vi "D_Datagrid example.vi"(10 "Remote stop event":refnum<user-event>, 11 "Owning VI":refnum<vi>) -> ()   [LabVIEW 2023, in "D Datagrid Library.lvlib"]
uses:
  D Datagrid Library.lvlib
  Scrolling behavior.ctl
  U32 D Element/U32 D Element.lvclass
  U8 D Element/U8 D Element.lvclass
  Bool D Element/Bool D Element.lvclass
  U32 D Element/Display mode.ctl
  String Dropdown D Element/String dropdown D Element.lvclass
  COM port D Element/COM Port D Element.lvclass
  D_Datagrid.lvclass
  String D Element/String D Element.lvclass
  String Dropdown D Element/String dropdown D Element.lvclass/String dropdown D Element.ctl
  U8 D Element/U8 D Element.lvclass/U8 D Element.ctl
  String D Element/String D Element.lvclass/String D Element.ctl
  DatagridElement/DatagridElement.lvclass/DatagridElement.ctl
  Bool D Element/Bool D Element.lvclass/Bool D Element.ctl
  D_Datagrid.lvclass/D_Datagrid.ctl
  Write Auto update indicator.vi
  Bool D Element/Write F string.vi
  Bool D Element/Write T string.vi
  String Dropdown D Element/Write value.vi
  String Dropdown D Element/Write Strings.vi
  U8 D Element/Write Display mode.vi
  String D Element/Write Value.vi
  DatagridElement/Write Enabled state.vi
  Read Auto update indicator.vi
  DatagridElement/DatagridElement.lvclass
  C:/dev/D Datagrid/DatagridElement/DatagridElement.lvclass
  C:/dev/D Datagrid/String D Element/String D Element.lvclass
  C:/dev/D Datagrid/Bool D Element/Bool D Element.lvclass
  C:/dev/D Datagrid/U32 D Element/U32 D Element.lvclass
  C:/dev/D Datagrid/U8 D Element/U8 D Element.lvclass
  C:/dev/D Datagrid/String Dropdown D Element/String dropdown D Element.lvclass
  C:/dev/D Datagrid/COM port D Element/COM Port D Element.lvclass
panel:
  in  "Scrolling mode":T1
  in  "Update now":bool
  in  "Auto-update?":bool=TRUE
  out "New?":bool
  out "Data as string":string
  out "Column":i32
  out "Row":i32
  in  "Datagrid table":string[][](table)
  # "This is an optional input\nused if this VI is to be\ncalled from within a\nsubpanel."
  # "This event stops\nthe VI (if used\nin subpanel)"
  # "Element touched"
  # "Instructions:\n1- Run the VI.\n2- Click each cell. Disabled string and Grayed string\n     cannot be edited, but the rest can.\n3. Observe the Element Touched event information."
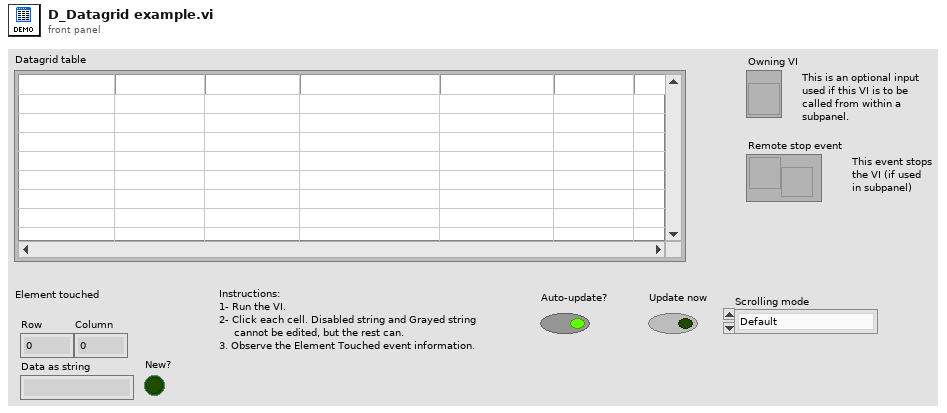
[diagram p1: front panel]
types:
  T1 = typedef "D Datagrid Library.lvlib/D_Datagrid.lvclass/Scrolling behavior.ctl" = enum16{"Default", "Locked", "Displayed items only"}
  T2 = enum8{"Enabled", "Disabled", "Disabled and Grayed Out"}
  T3 = typedef "D Datagrid Library.lvlib/U32 D Element.lvclass/Display mode.ctl" = enum16{"Standard", "Hex"}
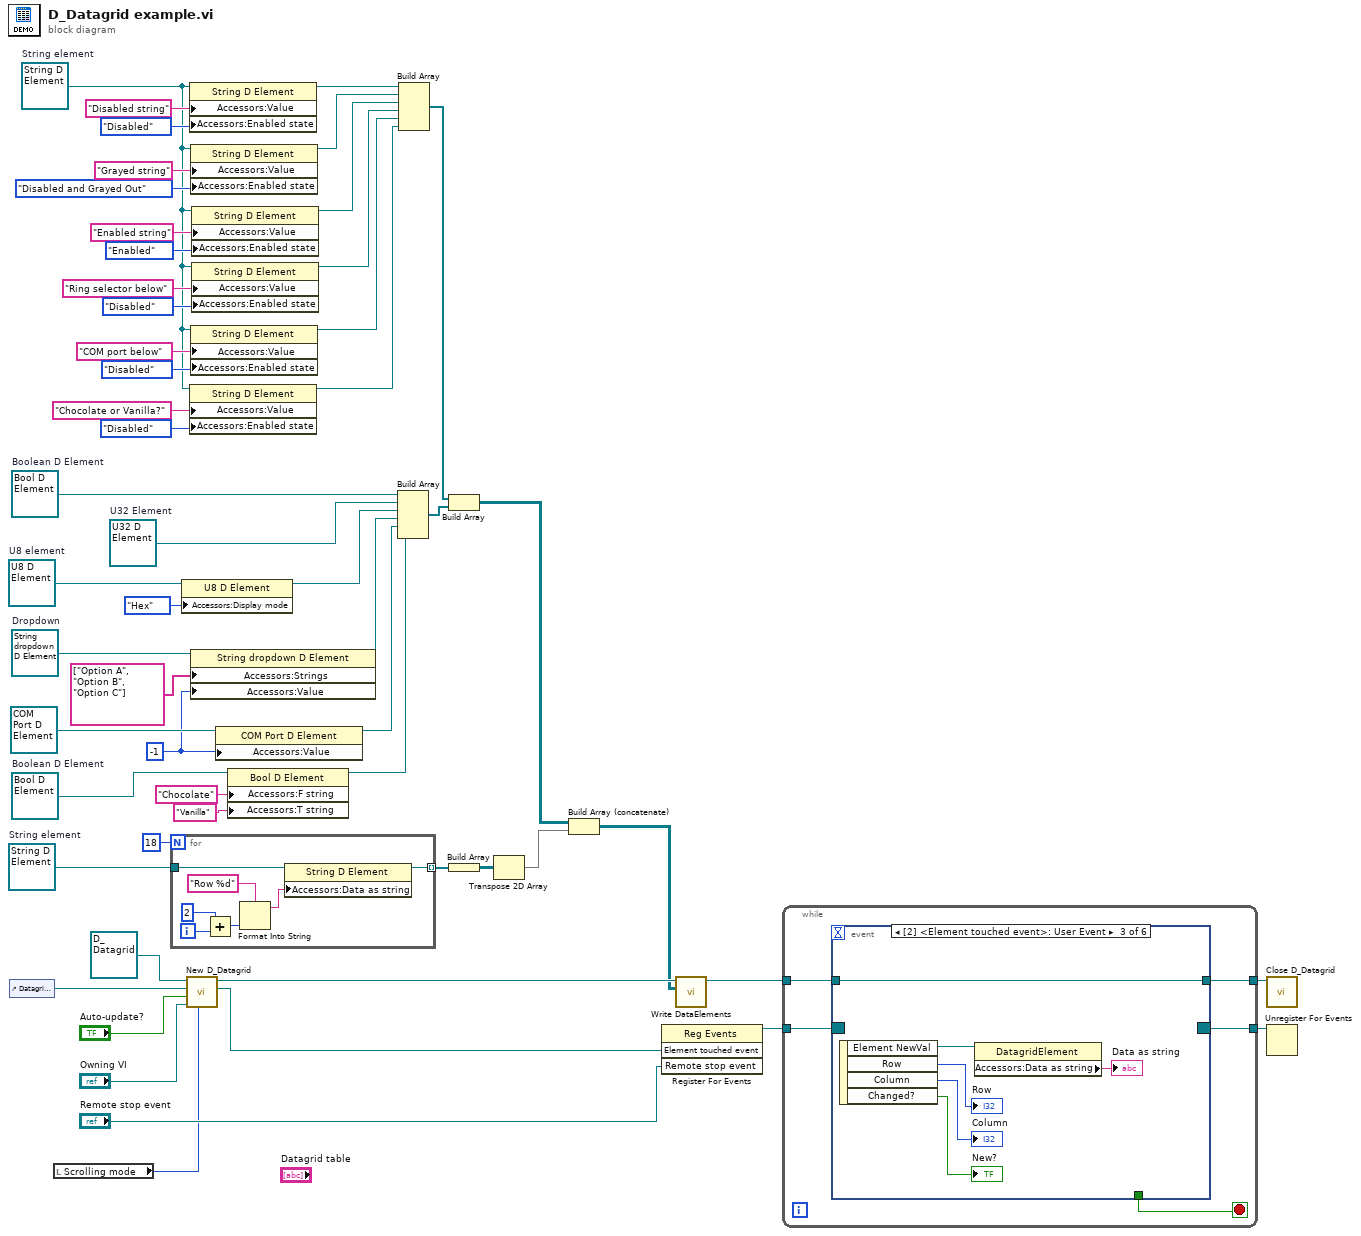
[diagram p0: block diagram]
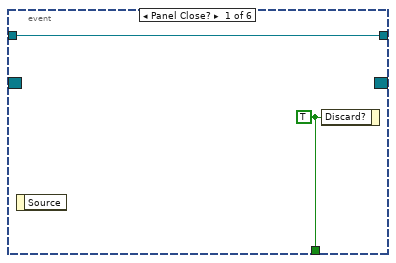
[diagram p2: hidden frame]
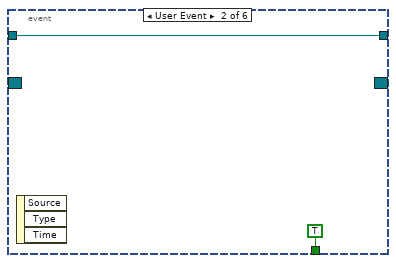
[diagram p3: hidden frame]
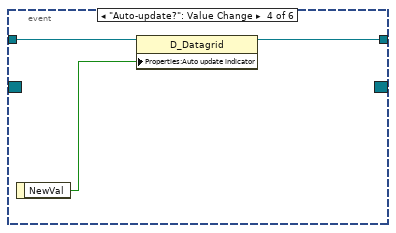
[diagram p4: hidden frame]
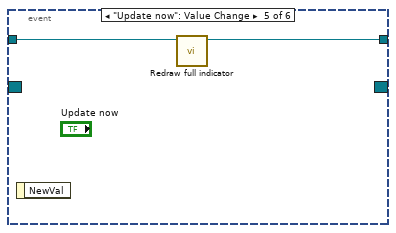
[diagram p5: hidden frame]
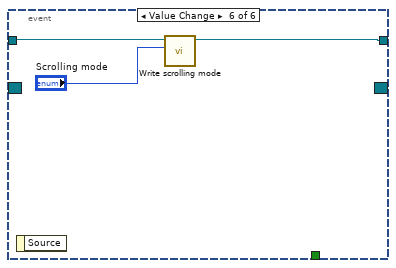
[diagram p6: hidden frame]
diagram:
  w8 = refnum<class "String D Element.lvclass"> refnum  # String element
  w14 = refnum<class "Bool D Element.lvclass"> refnum  # Boolean D Element
  w21 = -1 ("Value")
  w29 = refnum<class "String dropdown D Element.lvclass"> refnum  # Dropdown
  w38 = refnum<class "Bool D Element.lvclass"> refnum  # Boolean D Element
  w40 = refnum<class "U8 D Element.lvclass"> refnum  # U8 element
  w37 = refnum<class "U32 D Element.lvclass"> refnum  # U32 Element
  w9 = refnum<class "String D Element.lvclass"> refnum  # String element
  n1 = control-ref of="Datagrid table"() -> (w55:refnum<vi>)
  n2 = local read "Scrolling mode"() -> (w1:T1)
  n3 = for {
    N: 18 -> [_]
    tunnel: w8 -> [w62]
    tunnel: [w61] -> w6 mode=indexing
    i -> [w59]
    n4 = Add(x=2, y=w59) -> (x+y=w57:i32)
    n5 = Format Into String(format string="Row %d", w57) -> (resulting string=w56:string)  [unwired: 2 in, 1 out]
    n6 = property class="String D Element"(reference=w62, "Accessors:Data as string"=w56) -> (reference out=w61:refnum<class "String D Element.lvclass">)  [unwired: 1 in, 1 out]
  }
  n7 = property class="U8 D Element"(reference=w40, "Accessors:Display mode"=Display_mode."Hex" ("Display mode")) -> (reference out=w36:refnum<class "U8 D Element.lvclass">)  [unwired: 1 in, 1 out]
  n8 = call-dynamic "New D_Datagrid.vi"("Scrolling mode (default)"=w1, "Owning VI (caller)"="Owning VI", "Auto update indicator? (T)"="Auto-update?", "Indicator reference"=w55, "D_Datagrid in"=refnum<class "D_Datagrid.lvclass"> refnum) -> ("Element touched event"=w51:refnum<user-event>, "D_Datagrid out"=w54:refnum<class "D_Datagrid.lvclass">)  [unwired: 3 in, 2 out]
  n9 = property class="String D Element"(reference=w9, "Accessors:Value"="Disabled string" ("Value"), "Accessors:Enabled state"=T2."Disabled" ("Enabled state")) -> (reference out=w42:refnum<class "String D Element.lvclass">)  [unwired: 1 in, 1 out]
  n10 = property class="String D Element"(reference=w9, "Accessors:Value"="Chocolate or Vanilla?" ("Value"), "Accessors:Enabled state"=T2."Disabled" ("Enabled state")) -> (reference out=w10:refnum<class "String D Element.lvclass">)  [unwired: 1 in, 1 out]
  n11 = property class="String D Element"(reference=w9, "Accessors:Value"="Grayed string" ("Value"), "Accessors:Enabled state"=T2."Disabled and Grayed Out" ("Enabled state")) -> (reference out=w41:refnum<class "String D Element.lvclass">)  [unwired: 1 in, 1 out]
  n12 = property class="String D Element"(reference=w9, "Accessors:Value"="COM port below" ("Value"), "Accessors:Enabled state"=T2."Disabled" ("Enabled state")) -> (reference out=w25:refnum<class "String D Element.lvclass">)  [unwired: 1 in, 1 out]
  n13 = property class="String dropdown D Element"(reference=w29, "Accessors:Strings"=string[] ["Option A", "Option B", "Option C"] ("Strings"), "Accessors:Value"=w21) -> (reference out=w28:refnum<class "String dropdown D Element.lvclass">)  [unwired: 1 in, 1 out]
  n14 = property class="String D Element"(reference=w9, "Accessors:Value"="Enabled string" ("Value"), "Accessors:Enabled state"=T2."Enabled" ("Enabled state")) -> (reference out=w33:refnum<class "String D Element.lvclass">)  [unwired: 1 in, 1 out]
  n15 = property class="String D Element"(reference=w9, "Accessors:Value"="Ring selector below" ("Value"), "Accessors:Enabled state"=T2."Disabled" ("Enabled state")) -> (reference out=w30:refnum<class "String D Element.lvclass">)  [unwired: 1 in, 1 out]
  n16 = property class="COM Port D Element"(reference=refnum<class "COM Port D Element.lvclass"> refnum ("D Datagrid Library.lvlib:COM Port D Element"), "Accessors:Value"=w21) -> (reference out=w22:refnum<class "COM Port D Element.lvclass">)  [unwired: 1 in, 1 out]
  n17 = property class="Bool D Element"(reference=w14, "Accessors:F string"="Chocolate" ("F string"), "Accessors:T string"="Vanilla" ("F string")) -> (reference out=w11:refnum<class "Bool D Element.lvclass">)  [unwired: 1 in, 1 out]
  n18 = Build Array(w38, w37, w36, w28, w22, w11) -> (w35:refnum<class "DatagridElement.lvclass">[])
  n19 = Build Array(w42, w41, w33, w30, w25, w10) -> (w34:refnum<class "String D Element.lvclass">[])
  n20 = Build Array(w34, w35) -> (w3:refnum<class "DatagridElement.lvclass">[][])
  n21 = Build Array(w6) -> (w5:refnum<class "String D Element.lvclass">[][])
  n22 = Transpose 2D Array(2D array=w5) -> (transposed array=w4:refnum<class "String D Element.lvclass">[][])
  n23 = Build Array (concatenate)(w3, w4) -> (w2:refnum<class "DatagridElement.lvclass">[][])
  n24 = register-events(w51, "Remote stop event") -> (reference out=w50:refnum<event-registration>)  [unwired: 2 in, 1 out]
  n25 = call "Write DataElements.vi"("Data elements"=w2, "D_Datagrid in"=w54) -> ("D_Datagrid out"=w53:refnum<class "D_Datagrid.lvclass">)  [unwired: 8 in, 1 out]
  n26 = while {
    tunnel: w53 -> [w66]
    tunnel: [w65] -> w52
    tunnel: w50 -> [w64]
    tunnel: [w63] -> w49
    stop <- w67 stop-if-true
    n27 = event shown="[2] <Element touched event>: User Event" {
      selector: w64 -> [_ _ _ _ _ _]
      dyn-events: [_ _ _ _ _ _] -> w63
      timeout: _ -> [_ _ _ _ _ _]
      tunnel: [w69 TRUE ("Discard?") _ _ _ _] -> w67
      tunnel: w66 -> [w68 w71 w76 w80 w82 w85]
      tunnel: [w68 w71 w76 w79 w81 w83] -> w65
      event Panel Close? {
        w69 = TRUE ("Discard?")
        n28 = event-data() -> ()  [unwired: 1 in, 1 out]
        n29 = event-data("Discard?"=w69) -> ()  [unwired: 1 in, 1 out]
      }
      event User Event {
        n30 = event-data() -> ()  [unwired: 1 in, 3 out]
      }
      event User Event {
        n31 = event-data() -> ("Element NewVal"=w73:refnum<class "DatagridElement.lvclass">, "Row"=→"Row":i32, "Column"=→"Column":i32, "Changed?"=→"New?":bool)  [unwired: 1 in]
        n32 = property class="DatagridElement"(reference=w73) -> ("Accessors:Data as string"=→"Data as string":string)  [unwired: 1 in, 2 out]
      }
      event "Auto-update?": Value Change {
        n33 = event-data() -> ("NewVal"=w78:bool)  [unwired: 1 in]
        n34 = property class="D_Datagrid"(reference=w80, "Properties:Auto update indicator"=w78) -> (reference out=w79:refnum<class "D_Datagrid.lvclass">)  [unwired: 1 in, 1 out]
      }
      event "Update now": Value Change {
        n35 = event-data() -> ()  [unwired: 1 in, 1 out]
        n36 = call "Redraw full indicator.vi"("D_Datagrid in"=w82) -> ("D_Datagrid out"=w81:refnum<class "D_Datagrid.lvclass">)  [unwired: 9 in, 1 out]
      }
      event Value Change {
        n37 = event-data() -> ()  [unwired: 1 in, 1 out]
        n38 = call "Write scrolling mode.vi"("Scrolling mode"="Scrolling mode", "D_Datagrid in"=w85) -> ("D_Datagrid out"=w83:refnum<class "D_Datagrid.lvclass">)  [unwired: 8 in, 1 out]
      }
    }
  }
  n39 = call "Close D_Datagrid.vi"("D_Datagrid in"=w52) -> ()  [unwired: 10 in, 1 out]
  n40 = Unregister For Events(event registration refnum=w49) -> ()  [unwired: 1 in, 1 out]
